vi "convert_string_to_stringsArray.vi"(2 "Max Elements Count (All)":i32=-1, 4 "String in":string) -> (0 "string array size out":i32, 1 "string array out":string[](array[string]))   [LabVIEW 2020, in "Rohde&Schwarz RTx Oscilloscopes.lvlib" / "rsidr_core.lvlib"]
uses:
  rsidr_core.lvlib
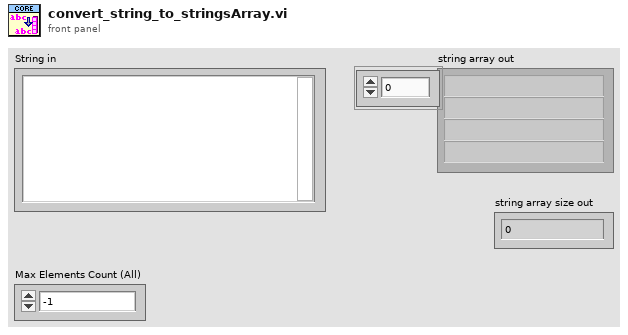
[diagram p1: front panel]
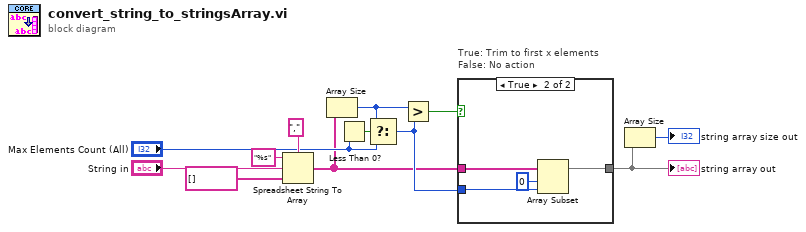
[diagram p0: block diagram]
diagram:
  n1 = Spreadsheet String To Array(delimiter (Tab)=",", format string="%s", spreadsheet string="String in", array type (2D Dbl)=string[] []) -> (array=w2:string[])
  n2 = Array Size(array=w2) -> (size(s)=w6:i32)
  n3 = Less Than 0?(x="Max Elements Count (All)") -> (x < 0?=w7:bool)
  n4 = Select(t=w6, s=w7, f="Max Elements Count (All)") -> (s? t:f=w3:i32)
  n5 = Greater?(x=w6, y=w3) -> (0:w5:bool)
  n6 = case "True: Trim to first x elements\nFalse: No action" shown="True" w5 {
    tunnel: w2 -> [w13 w17]
    tunnel: w3 -> [_ w15]
    tunnel: [w13 w14] -> w1
    frame False {
    }
    frame True {
      n7 = Array Subset(array=w17, index=0, length=w15) -> (w14:string[])
    }
  }
  "string array out" <- w1
  n8 = Array Size(array=w1) -> (size(s)=→"string array size out":i32)
